vi "Main.vi"() -> ()   [LabVIEW 2017]
doc: "Le programme Main est l'IHM principal du programme MonoSelector. Il controle le sélecteur d'onde de la manipe \"FastFlim\". Il acquit le spectre du laser et permet de positioner le sélecteur ainsi que de choisir la bande passante des ondes lumineuse."
uses:
  Lib IHM Control/MHL Data.ctl
  Lib IHM Control/MHL UI Data.ctl
  <vilib>/vision/Image Controls.llb/IMAQ Image.ctl
  Lib IHM Control/MHL UI Ref.ctl
  Lib IHM Control/Front Panel Status.ctl
  Lib QMH/MessageQueues.lvlib
  Lib Notifier/Notifier.lvlib
  Lib IHM Control/IHM Control.lvlib
  Lib Log/Logging.lvlib
panel:
  in  "Pulse Picker Set":u16(ring) items=["80"=80, "40"=40, "20"=20]
  out "Laser Connection":bool
  out "Camera":T1(plugin-control)
  in  "Integration (ms)":i32=100
  in  "Stop":bool
  in  "View":bool
  in  "LaserON":bool
  out "Power":dbl
  in  "LaserOFF":bool
  out "Pulse Picker":dbl
  in  "Power Set":dbl=480.0
  out "StedFLIM Status":string
  # "Laser"
  # "Camera"
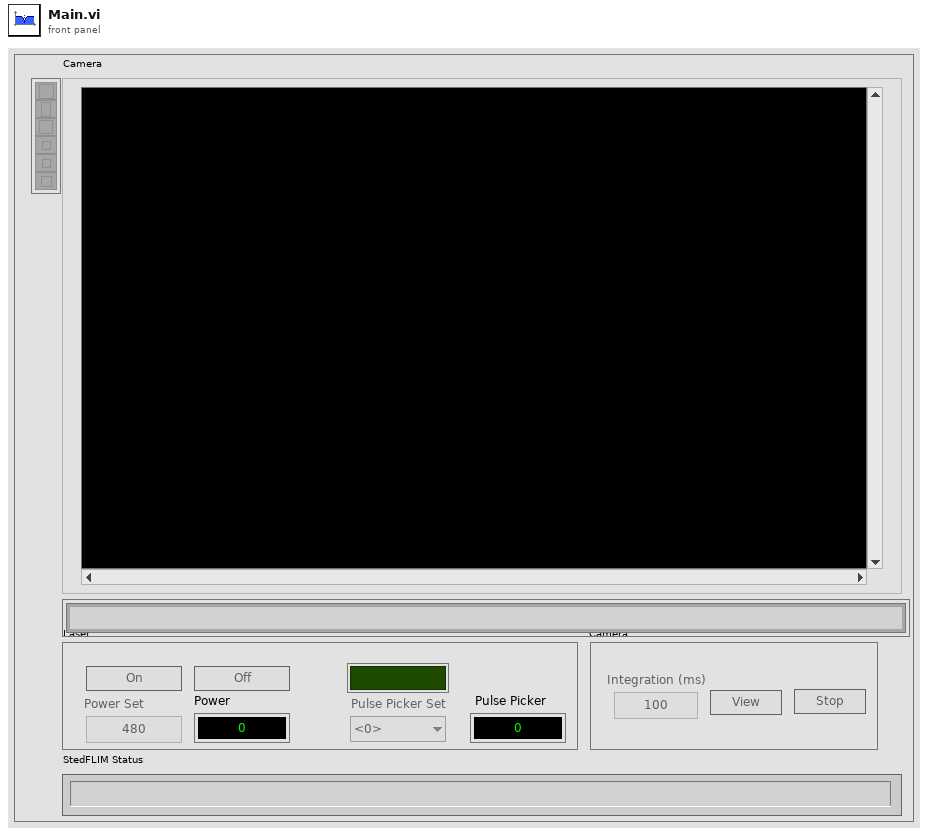
[diagram p1: front panel]
types:
  T1 = typedef "IMAQ Image.ctl" = refnum<image>
  T2 = typedef "MHL Data.ctl" = cluster{"IHM Data":T3, "MHL ref":T4, "Front Panel status":T5}
  T3 = typedef "MHL UI Data.ctl" = cluster{"Integration":i32, "Set Power":dbl, "Power":dbl, "Set Pulse Picke":dbl, "Pulse Picker":dbl, "Status StedFLIM":string, "View":T1, "Laser Connection":bool}
  T4 = typedef "IHM Control.lvlib/MHL UI Ref.ctl" = cluster{"View":refnum<vi>, "Stop":refnum<vi>, "Laser OFF":refnum<vi>, "Laser ON":refnum<vi>, "Integration":refnum<vi>, "SetPower":refnum<vi>, "SetPulsePicker":refnum<vi>}
  T5 = typedef "IHM Control.lvlib/Front Panel Status.ctl" = enum16{"Initialisation", "Enable Laser", "Enable Camera", "Disable Laser", "Disable Camera"}
  T6 = typedef "MessageQueues.lvlib/AllMessageQueue Cluster.ctl" = cluster{"MHL":refnum<queue>, "Recipe":refnum<queue>, "Laser":refnum<queue>, "Laser Controller":refnum<queue>, "Camera":refnum<queue>, "Camera Controller":refnum<queue>, "Manager":refnum<queue>}
  T7 = typedef "Notifier.lvlib/Notifier.ctl" = cluster{"Camera Handshake":refnum<notifier>, "Camera Ctrl Exit":refnum<notifier>, "Camera Exit":refnum<notifier>, "Laser Hanshake":refnum<notifier>, "Laser Ctrl Exit":refnum<notifier>, "Laser Exit":refnum<notifier>}
  T8 = enum16{"open", "replace", "create", "open or create", "replace or create", "replace or create with confirmation"}
  T9 = cluster{"état":bool, "code":i32, "source":string}
  T10 = enum32{"Invalid", "Standard", "Closed", "Hidden", "Minimized", "Maximized"}
  T11 = enum32{"invalid app kind", "Development System", "Run Time System", "Student Edition", "Embedded LabVIEW", "Evaluation", "Custom"}
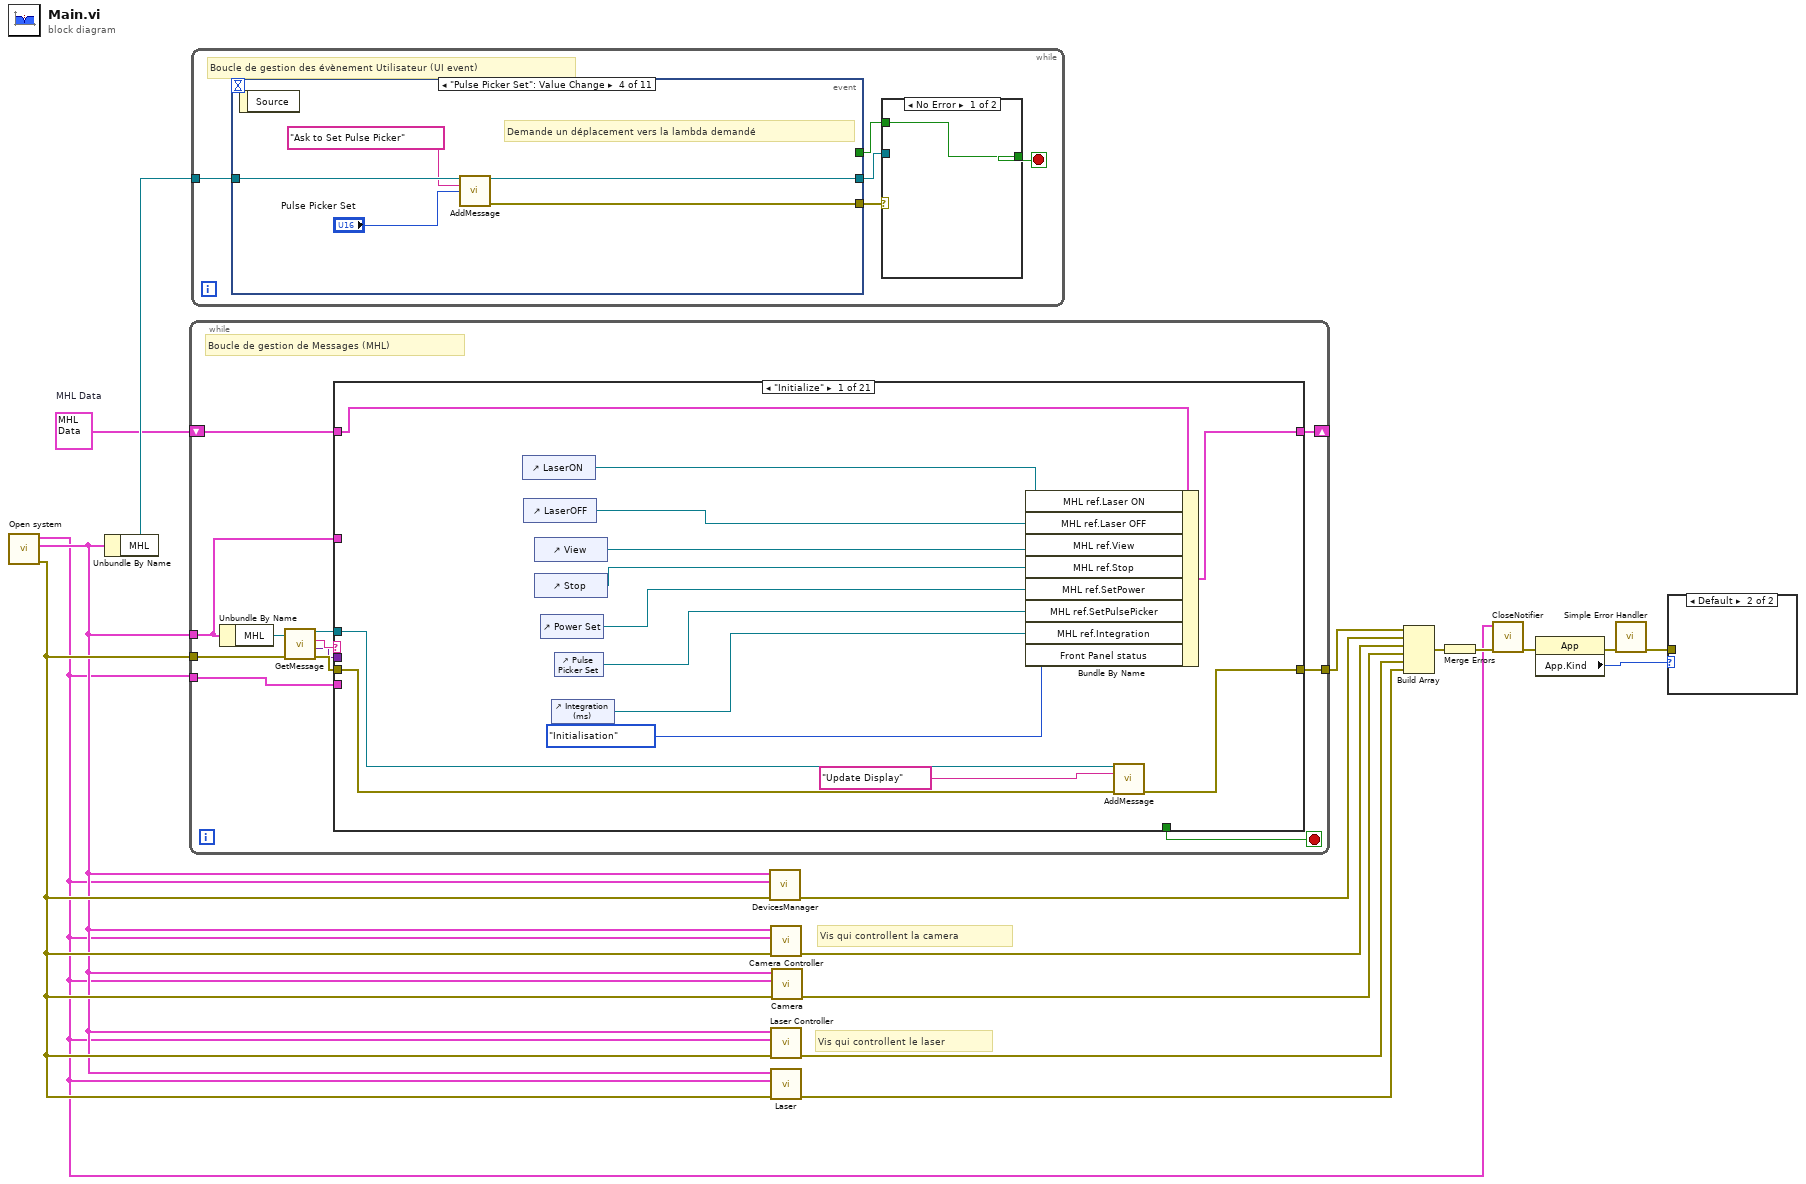
[diagram p0: block diagram]
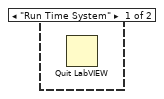
[diagram p2: hidden frame]
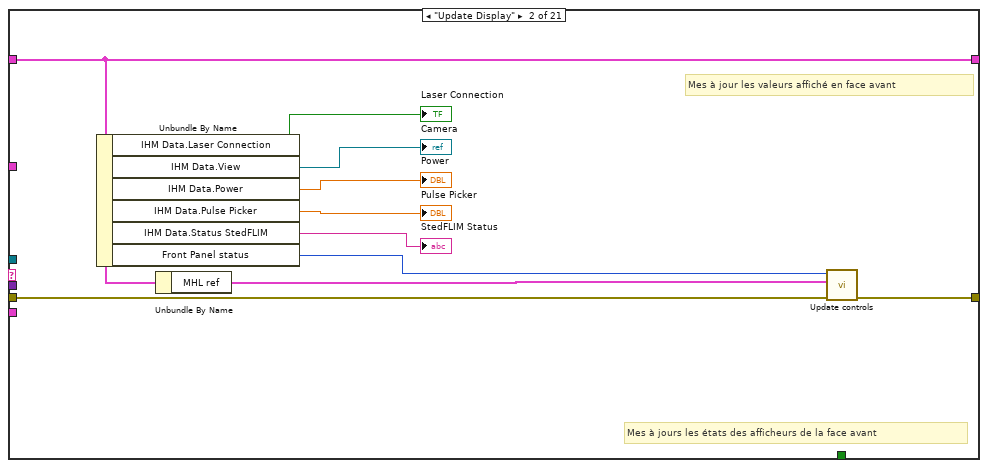
[diagram p3: hidden frame]
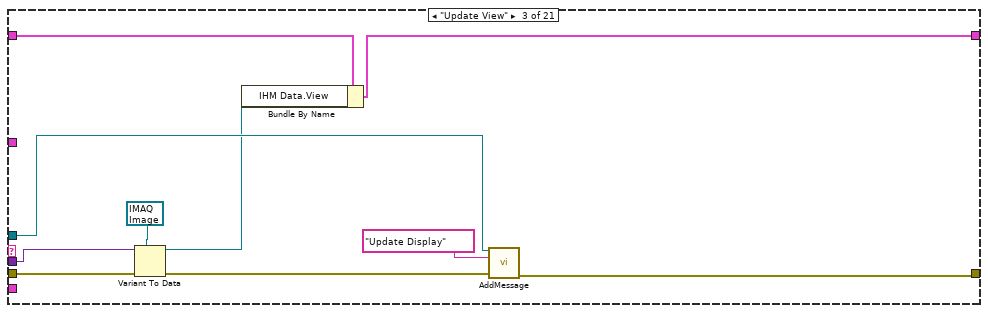
[diagram p4: hidden frame]
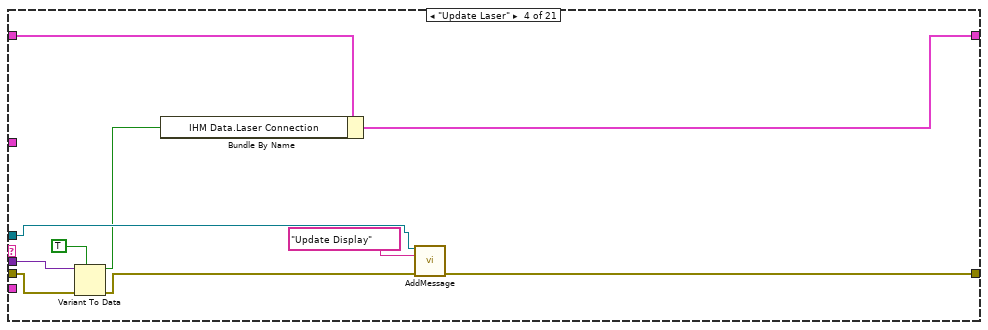
[diagram p5: hidden frame]
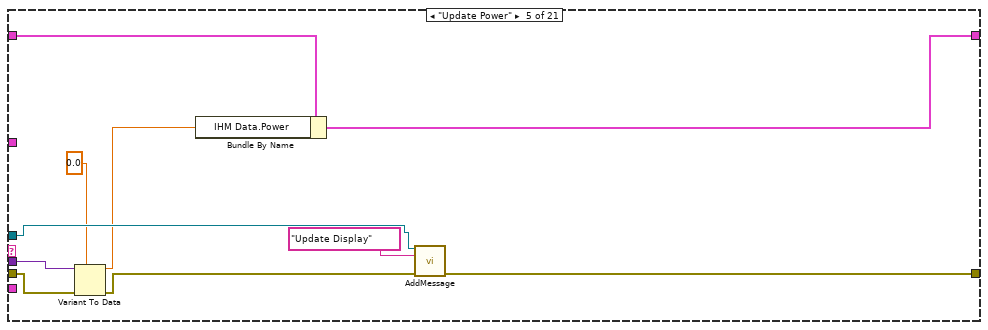
[diagram p6: hidden frame]
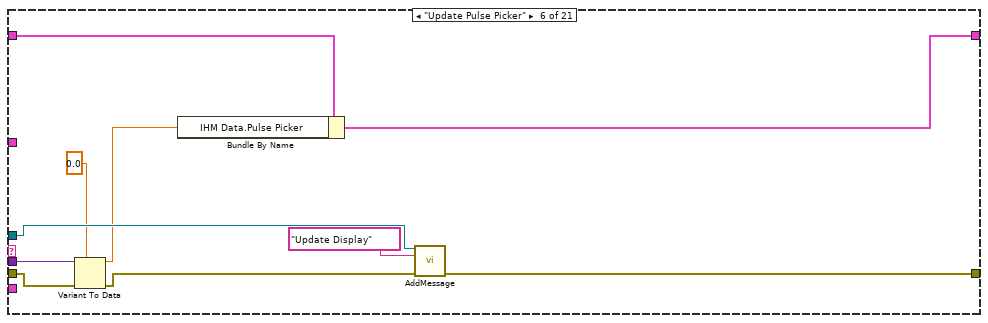
[diagram p7: hidden frame]
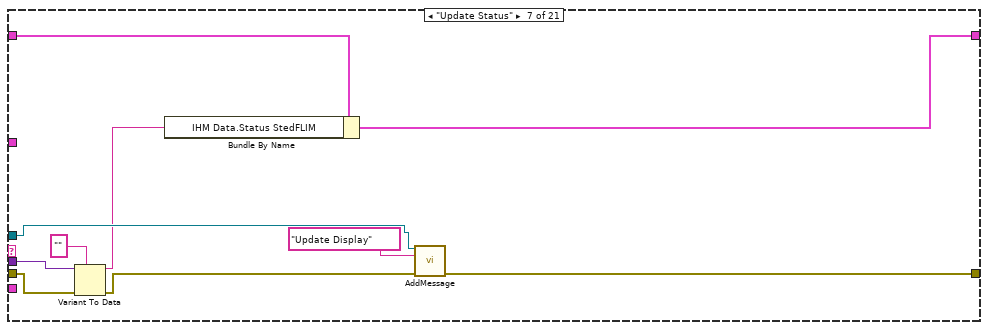
[diagram p8: hidden frame]
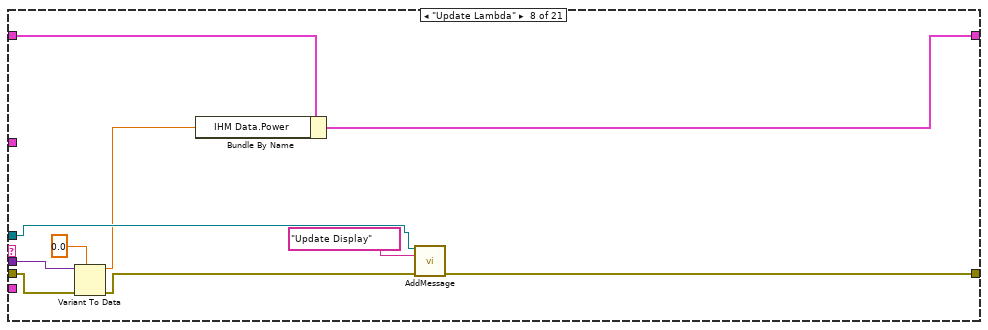
[diagram p9: hidden frame]
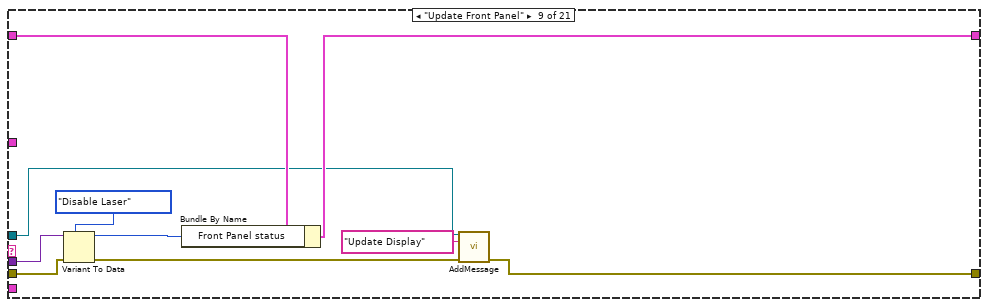
[diagram p10: hidden frame]
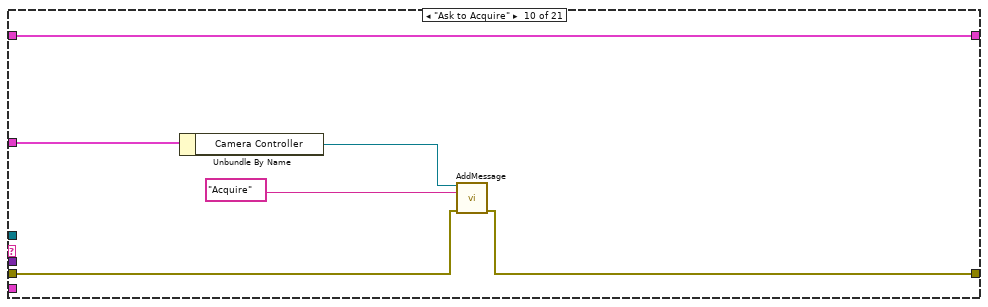
[diagram p11: hidden frame]
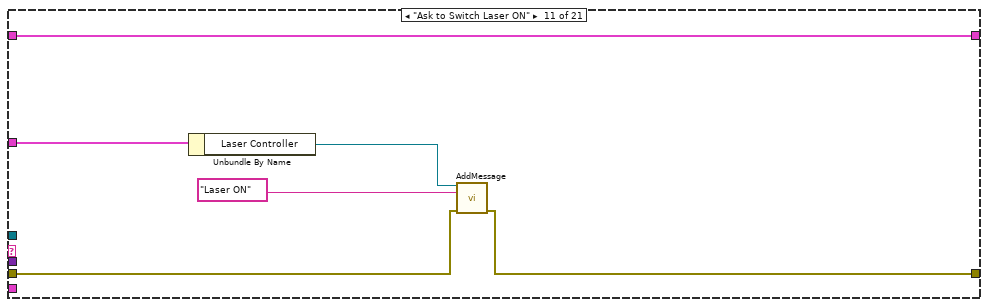
[diagram p12: hidden frame]
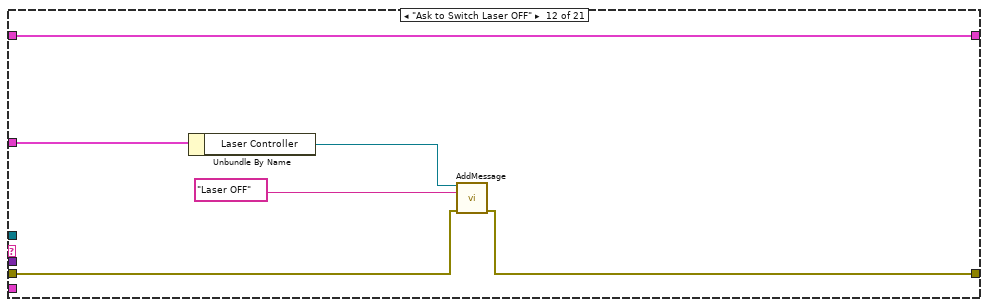
[diagram p13: hidden frame]
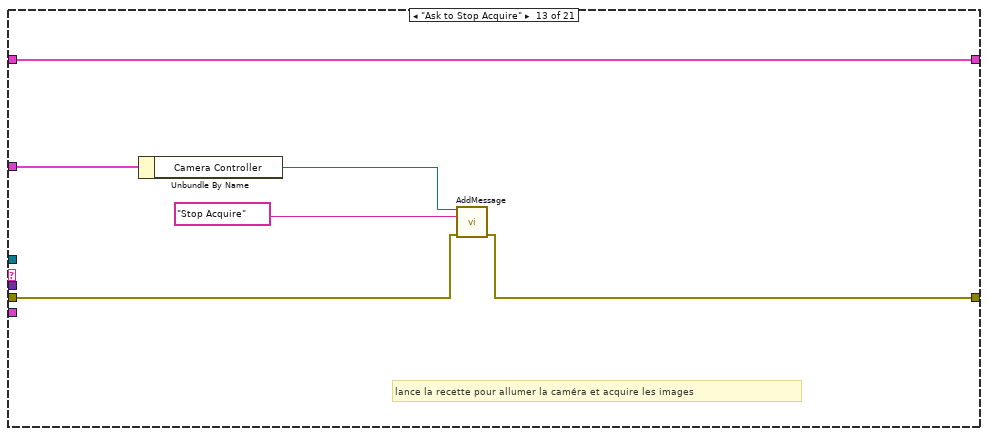
[diagram p14: hidden frame]
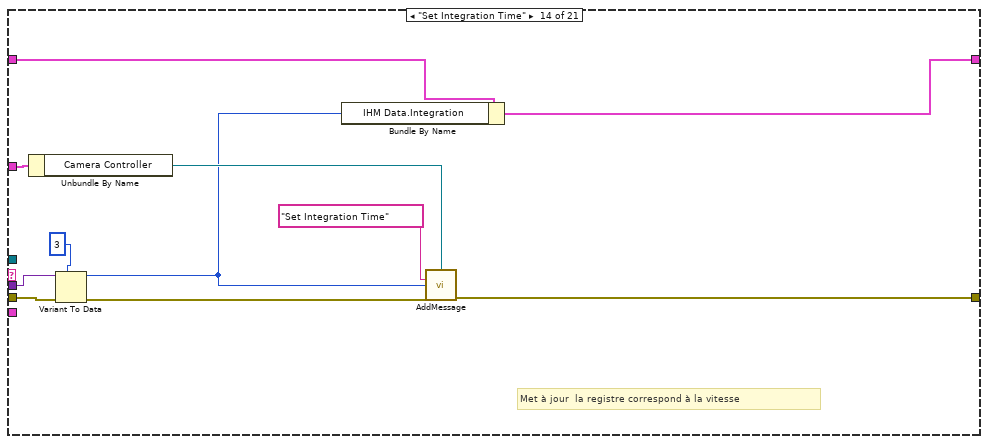
[diagram p15: hidden frame]
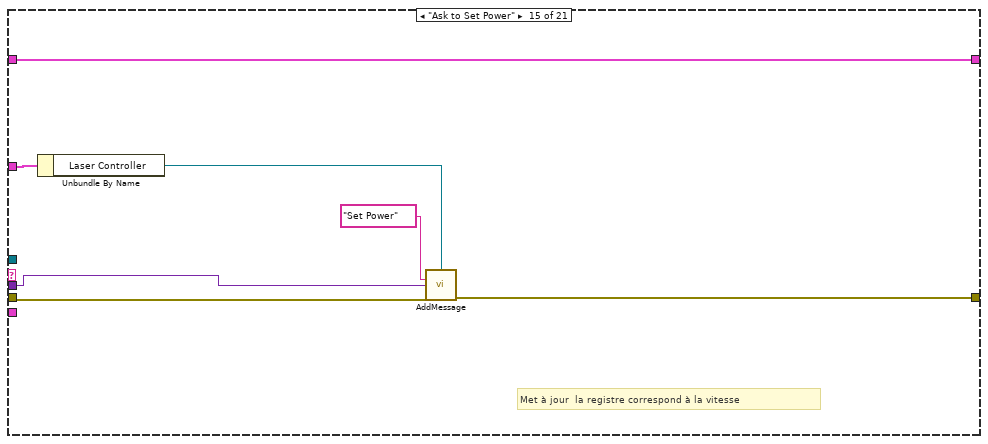
[diagram p16: hidden frame]
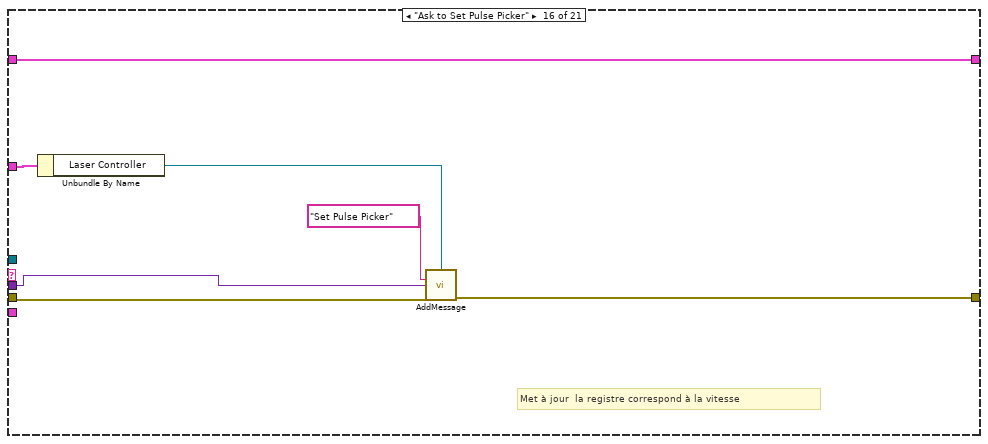
[diagram p17: hidden frame]
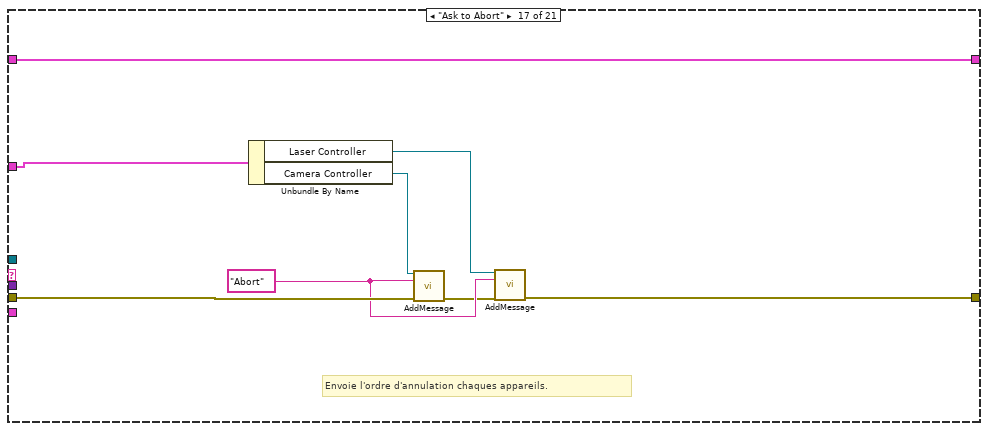
[diagram p18: hidden frame]
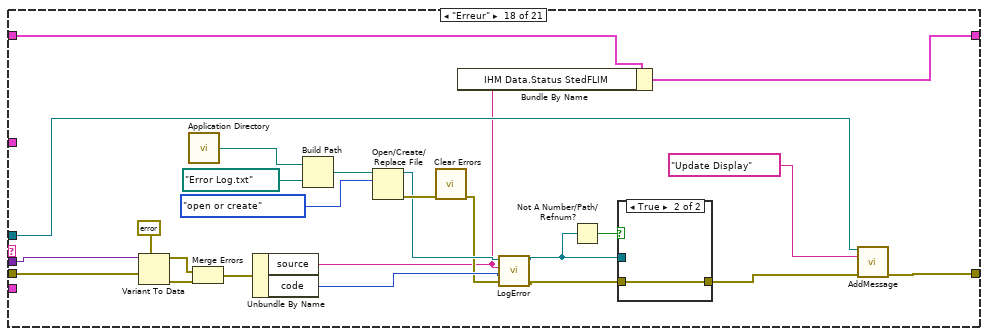
[diagram p19: hidden frame]
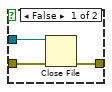
[diagram p20: hidden frame]
diagram:
  w10 = T2 {"IHM Data"={"Integration"=0, "Set Power"=0.0, "Power"=0.0, "Set Pulse Picke"=0.0, "Pulse Picker"=0.0, "Status StedFLIM"="", "View"=refnum, "Laser Connection"=FALSE}, "MHL ref"={"View"=refnum, "Stop"=refnum, "Laser OFF"=refnum, "Laser ON"=refnum, "Integration"=refnum, "SetPower"=refnum, "SetPulsePicker"=refnum}, "Front Panel status"=enum."Initialisation"}  # MHL Data
  # "Vis qui controllent le laser"
  # "Vis qui controllent la camera"
  n1 = call "Open system.vi"() -> ("error out"=w5:errorcluster, "All Message Queue Cluster"=w2:T6, "Notifiers"=w1:T7)  [unwired: 8 in, 1 out]
  n2 = Unbundle By Name(w2) -> ("MHL"=w13:refnum<queue>)
  n3 = while {
    tunnel: w1 -> [w27]
    tunnel: w2 -> [w26]
    shift-right: [w18] -> _
    shift-left: w10 -> [w19]
    tunnel: w5 -> [w24]
    tunnel: [w29] -> w4
    stop <- w28 stop-if-true
    # "Boucle de gestion de Messages (MHL)"
    n4 = Unbundle By Name(w26) -> ("MHL"=w25:refnum<queue>)
    n5 = call "GetMessage.vi"("entrée d'erreur"=w24, "Message queue"=w25) -> ("sortie d'erreur"=w23:errorcluster, "Data"=w20:variant, "Message"=w21:string, "Dup Message Queue"=w22:refnum<queue>)  [unwired: 6 in]
    n6 = case shown="\"Initialize\"" w21 {
      tunnel: w26 -> [_ _ _ _ _ _ _ _ _ w129 w135 w141 w147 w157 w164 w171 w180 _ _ _ w228]
      tunnel: w22 -> [w39 _ w57 w71 w81 w91 w101 w111 w115 _ _ _ _ _ _ _ _ w185 _ w215 _]
      tunnel: w23 -> [w41 w53 w62 w68 w79 w89 w98 w108 w123 w126 w132 w138 w144 w153 w160 w167 w177 w194 w211 w214 w217]
      tunnel: [w40 w52 w58 w72 w82 w92 w102 w112 w116 w125 w131 w137 w143 w158 w165 w172 w173 w186 w211 w213 w220] -> w29
      tunnel: [_ _ _ _ _ _ _ _ _ _ _ _ _ _ _ _ _ _ _ TRUE _] -> w28
      tunnel: w27 -> [_ _ _ _ _ _ _ _ _ _ _ _ _ _ _ _ _ _ _ _ _]
      tunnel: w20 -> [_ _ w61 w70 w80 w90 w100 w110 w122 _ _ _ _ w151 w161 w168 _ w193 _ _ _]
      tunnel: w19 -> [w43 w50 w63 w66 w77 w87 w96 w106 w120 w124 w130 w136 w142 w154 w159 w166 w178 w184 w209 w212 w227]
      tunnel: [w42 w50 w56 w65 w76 w86 w95 w105 w118 w124 w130 w136 w142 w148 w159 w166 w178 w181 w209 w212 w227] -> w18
      frame "Initialize" {
        n7 = control-ref of="LaserON"() -> (w31:refnum<vi>)
        n8 = control-ref of="LaserOFF"() -> (w32:refnum<vi>)
        n9 = control-ref of="View"() -> (w33:refnum<vi>)
        n10 = control-ref of="Stop"() -> (w34:refnum<vi>)
        n11 = control-ref of="Power Set"() -> (w35:refnum<vi>)
        n12 = control-ref of="Integration (ms)"() -> (w36:refnum<vi>)
        n13 = control-ref of="Pulse Picker Set"() -> (w30:refnum<vi>)
        n14 = Bundle By Name(cluster=w43, "MHL ref.Laser ON"=w31, "MHL ref.Laser OFF"=w32, "MHL ref.View"=w33, "MHL ref.Stop"=w34, "MHL ref.SetPower"=w35, "MHL ref.SetPulsePicker"=w30, "MHL ref.Integration"=w36, "Front Panel status"=Front_Panel_Status."Initialisation") -> (w42:T2)
        n15 = call "AddMessage.vi"("Message queue"=w39, "Message"="Update Display", "entrée d'erreur (pas d'erreur)"=w41) -> ("error out"=w40:errorcluster)  [unwired: 11 in, 1 out]
      }
      frame "Update Display" {
        # "Mes à jours les états des afficheurs de la face avant"
        # "Mes à jour les valeurs affiché en face avant"
        n16 = Unbundle By Name(w50) -> ("IHM Data.Laser Connection"=→"Laser Connection":bool, "IHM Data.View"=→"Camera":T1, "IHM Data.Power"=→"Power":dbl, "IHM Data.Pulse Picker"=→"Pulse Picker":dbl, "IHM Data.Status StedFLIM"=→"StedFLIM Status":string, "Front Panel status"=w49:T5)
        n17 = Unbundle By Name(w50) -> ("MHL ref"=w51:T4)
        n18 = call "Update controls.vi"("error in (no error)"=w53, "IHM Data refnum"=w51, "Front Panel status"=w49) -> ("error out"=w52:errorcluster)  [unwired: 8 in]
      }
      frame "Update View" {
        n19 = Variant To Data(error in=w62, type=T1 refnum ("IHM Data.View"), Variant=w61) -> (data=w54:T1, error out=w59:errorcluster)
        n20 = Bundle By Name(cluster=w63, "IHM Data.View"=w54) -> (w56:T2)
        n21 = call "AddMessage.vi"("Message queue"=w57, "Message"="Update Display", "entrée d'erreur (pas d'erreur)"=w59) -> ("error out"=w58:errorcluster)  [unwired: 11 in, 1 out]
      }
      frame "Update Laser" {
        n22 = Variant To Data(error in=w68, type=TRUE, Variant=w70) -> (data=w64:bool, error out=w67:errorcluster)
        n23 = Bundle By Name(cluster=w66, "IHM Data.Laser Connection"=w64) -> (w65:T2)
        n24 = call "AddMessage.vi"("Message queue"=w71, "Message"="Update Display", "entrée d'erreur (pas d'erreur)"=w67) -> ("error out"=w72:errorcluster)  [unwired: 11 in, 1 out]
      }
      frame "Update Power" {
        n25 = Variant To Data(error in=w79, type=0.0, Variant=w80) -> (data=w74:dbl, error out=w78:errorcluster)
        n26 = Bundle By Name(cluster=w77, "IHM Data.Power"=w74) -> (w76:T2)
        n27 = call "AddMessage.vi"("Message queue"=w81, "Message"="Update Display", "entrée d'erreur (pas d'erreur)"=w78) -> ("error out"=w82:errorcluster)  [unwired: 11 in, 1 out]
      }
      frame "Update Pulse Picker" {
        n28 = Variant To Data(error in=w89, type=0.0, Variant=w90) -> (data=w84:dbl, error out=w88:errorcluster)
        n29 = Bundle By Name(cluster=w87, "IHM Data.Pulse Picker"=w84) -> (w86:T2)
        n30 = call "AddMessage.vi"("Message queue"=w91, "Message"="Update Display", "entrée d'erreur (pas d'erreur)"=w88) -> ("error out"=w92:errorcluster)  [unwired: 11 in, 1 out]
      }
      frame "Update Status" {
        n31 = Variant To Data(error in=w98, type="", Variant=w100) -> (data=w94:string, error out=w97:errorcluster)
        n32 = Bundle By Name(cluster=w96, "IHM Data.Status StedFLIM"=w94) -> (w95:T2)
        n33 = call "AddMessage.vi"("Message queue"=w101, "Message"="Update Display", "entrée d'erreur (pas d'erreur)"=w97) -> ("error out"=w102:errorcluster)  [unwired: 11 in, 1 out]
      }
      frame "Update Lambda" {
        n34 = Variant To Data(error in=w108, type=0.0, Variant=w110) -> (data=w104:dbl, error out=w107:errorcluster)
        n35 = Bundle By Name(cluster=w106, "IHM Data.Power"=w104) -> (w105:T2)
        n36 = call "AddMessage.vi"("Message queue"=w111, "Message"="Update Display", "entrée d'erreur (pas d'erreur)"=w107) -> ("error out"=w112:errorcluster)  [unwired: 11 in, 1 out]
      }
      frame "Update Front Panel" {
        n37 = Variant To Data(error in=w123, type=Front_Panel_Status."Disable Laser" ("Front Panel status"), Variant=w122) -> (data=w119:T5, error out=w117:errorcluster)
        n38 = Bundle By Name(cluster=w120, "Front Panel status"=w119) -> (w118:T2)
        n39 = call "AddMessage.vi"("Message queue"=w115, "Message"="Update Display", "entrée d'erreur (pas d'erreur)"=w117) -> ("error out"=w116:errorcluster)  [unwired: 11 in, 1 out]
      }
      frame "Ask to Acquire" {
        n40 = Unbundle By Name(w129) -> ("Camera Controller"=w128:refnum<queue>)
        n41 = call "AddMessage.vi"("Message queue"=w128, "Message"="Acquire", "entrée d'erreur (pas d'erreur)"=w126) -> ("error out"=w125:errorcluster)  [unwired: 11 in, 1 out]
      }
      frame "Ask to Switch Laser ON" {
        n42 = Unbundle By Name(w135) -> ("Laser Controller"=w134:refnum<queue>)
        n43 = call "AddMessage.vi"("Message queue"=w134, "Message"="Laser ON", "entrée d'erreur (pas d'erreur)"=w132) -> ("error out"=w131:errorcluster)  [unwired: 11 in, 1 out]
      }
      frame "Ask to Switch Laser OFF" {
        n44 = Unbundle By Name(w141) -> ("Laser Controller"=w140:refnum<queue>)
        n45 = call "AddMessage.vi"("Message queue"=w140, "Message"="Laser OFF", "entrée d'erreur (pas d'erreur)"=w138) -> ("error out"=w137:errorcluster)  [unwired: 11 in, 1 out]
      }
      frame "Ask to Stop Acquire" {
        # "lance la recette pour allumer la caméra et acquire les images"
        n46 = Unbundle By Name(w147) -> ("Camera Controller"=w146:refnum<queue>)
        n47 = call "AddMessage.vi"("Message queue"=w146, "Message"="Stop Acquire", "entrée d'erreur (pas d'erreur)"=w144) -> ("error out"=w143:errorcluster)  [unwired: 11 in, 1 out]
      }
      frame "Set Integration Time" {
        # "Met à jour  la registre correspond à la vitesse"
        n48 = Unbundle By Name(w157) -> ("Camera Controller"=w156:refnum<queue>)
        n49 = Variant To Data(error in=w153, type=3 ("Integration (ms)"), Variant=w151) -> (data=w149:i32, error out=w152:errorcluster)
        n50 = Bundle By Name(cluster=w154, "IHM Data.Integration"=w149) -> (w148:T2)
        n51 = call "AddMessage.vi"("Message queue"=w156, "Message"="Set Integration Time", "Data"=w149, "entrée d'erreur (pas d'erreur)"=w152) -> ("error out"=w158:errorcluster)  [unwired: 10 in, 1 out]
      }
      frame "Ask to Set Power" {
        # "Met à jour  la registre correspond à la vitesse"
        n52 = Unbundle By Name(w164) -> ("Laser Controller"=w163:refnum<queue>)
        n53 = call "AddMessage.vi"("Message queue"=w163, "Message"="Set Power", "Data"=w161, "entrée d'erreur (pas d'erreur)"=w160) -> ("error out"=w165:errorcluster)  [unwired: 10 in, 1 out]
      }
      frame "Ask to Set Pulse Picker" {
        # "Met à jour  la registre correspond à la vitesse"
        n54 = Unbundle By Name(w171) -> ("Laser Controller"=w170:refnum<queue>)
        n55 = call "AddMessage.vi"("Message queue"=w170, "Message"="Set Pulse Picker", "Data"=w168, "entrée d'erreur (pas d'erreur)"=w167) -> ("error out"=w172:errorcluster)  [unwired: 10 in, 1 out]
      }
      frame "Ask to Abort" {
        w175 = "Abort" ("Message")
        # "Envoie l'ordre d'annulation chaques appareils."
        n56 = Unbundle By Name(w180) -> ("Laser Controller"=w176:refnum<queue>, "Camera Controller"=w179:refnum<queue>)
        n57 = call "AddMessage.vi"("Message queue"=w179, "Message"=w175, "entrée d'erreur (pas d'erreur)"=w177) -> ("error out"=w174:errorcluster)  [unwired: 11 in, 1 out]
        n58 = call "AddMessage.vi"("Message queue"=w176, "Message"=w175, "entrée d'erreur (pas d'erreur)"=w174) -> ("error out"=w173:errorcluster)  [unwired: 11 in, 1 out]
      }
      frame "Erreur" {
        n59 = Variant To Data(error in=w194, type=T9 {"état"=FALSE, "code"=0, "source"=""} ("sortie d'erreur"), Variant=w193) -> (data=w202:T9, error out=w203:errorcluster)
        n60 = call <vilib>:"Application Directory.vi"() -> ("Application Directory"=w200:path)
        n61 = Merge Errors(w202, w203) -> (w201:errorcluster)
        n62 = Unbundle By Name(w201) -> ("source"=w183:string, "code"=w190:i32)
        n63 = Build Path(base path=w200, name or relative path=path "Error Log.txt") -> (appended path=w199:path)
        n64 = Open/Create/Replace File(file path (use dialog)=w199, operation (0:open)=T8."open or create" ("opération (0 : open)")) -> (refnum out=w192:refnum<file>, error out=w195:errorcluster)  [unwired: 4 in, 1 out]
        n65 = call <vilib>:"Clear Errors.vi"("error in (no error)"=w195) -> ("error out"=w189:errorcluster)  [unwired: 5 in, 1 out]
        n66 = Bundle By Name(cluster=w184, "IHM Data.Status StedFLIM"=w183) -> (w181:T2)
        n67 = call "LogError.vi"("entrée d'erreur"=w189, "Code"=w190, "Source"=w183, "Error log refnum In"=w192) -> ("error out"=w188:errorcluster, "Error log refnum out"=w191:refnum<file>)  [unwired: 6 in]
        n68 = Not A Number/Path/Refnum?(number/path/refnum=w191) -> (NaN/Path/Refnum?=w196:bool)
        n69 = case shown="True" w196 {
          tunnel: w188 -> [w207 w208]
          tunnel: w191 -> [w206 _]
          tunnel: [w205 w208] -> w187
          frame False {
            n70 = Close File(refnum=w206, error in=w207) -> (error out=w205:errorcluster)  [unwired: 1 out]
          }
          frame True {
          }
        }
        n71 = call "AddMessage.vi"("Message queue"=w185, "Message"="Update Display", "entrée d'erreur (pas d'erreur)"=w187) -> ("error out"=w186:errorcluster)  [unwired: 11 in, 1 out]
      }
      frame Default {
        n72 = One Button Dialog(message="Warning : Message erroné ou erreur dans le MHL") -> ()  [unwired: 1 in, 1 out]
      }
      frame "Quit" {
        # "Libère la pile MHL et stop la boucle"
        n73 = Release Queue(queue=w215, error in (no error)=w214) -> (error out=w213:errorcluster)  [unwired: 1 in, 2 out]
      }
      frame "Initiate Stop" {
        w218 = "Exit" ("Message")
        # "Envoie un message d'arrête à tous les controleur.\nPuis demande d'attendre jusqu'à ce que chaque appareils soit arrêtés"
        n74 = Unbundle By Name(w228) -> ("MHL"=w219:refnum<queue>, "Laser Controller"=w226:refnum<queue>, "Camera Controller"=w225:refnum<queue>, "Manager"=w224:refnum<queue>)
        n75 = call "AddMessage.vi"("Message queue"=w225, "Message"=w218, "entrée d'erreur (pas d'erreur)"=w217) -> ("error out"=w222:errorcluster)  [unwired: 11 in, 1 out]
        n76 = call "AddMessage.vi"("Message queue"=w224, "Message"=w218, "entrée d'erreur (pas d'erreur)"=w217) -> ("error out"=w221:errorcluster)  [unwired: 11 in, 1 out]
        n77 = call "AddMessage.vi"("Message queue"=w226, "Message"=w218, "entrée d'erreur (pas d'erreur)"=w217) -> ("error out"=w223:errorcluster)  [unwired: 11 in, 1 out]
        n78 = Merge Errors(w223, w222, w221) -> (w220:errorcluster)
        n79 = case shown="No Error" w220 {
          selector: w220 -> [w229 _]
          tunnel: w219 -> [w231 _]
          frame No Error {
            n80 = call "AddMessage.vi"("Message queue"=w231, "Message"="Quit", "entrée d'erreur (pas d'erreur)"=w229) -> ()  [unwired: 11 in, 2 out]
          }
          frame Error {
          }
        }
      }
    }
  }
  n81 = while {
    tunnel: w13 -> [w236]
    stop <- w233 stop-if-true
    # "Boucle de gestion des évènement Utilisateur (UI event)"
    n82 = event shown="[3] \"Pulse Picker Set\": Value Change" {
      selector: _ -> [_ _ _ _ _ _ _ _ _ _ _]
      dyn-events: _ -> [_ _ _ _ _ _ _ _ _ _ _]
      timeout: _ -> [_ _ _ _ _ _ _ _ _ _ _]
      tunnel: w236 -> [_ w242 w250 w255 w259 w282 w288 w292 w297 w302 w307]
      tunnel: [_ w243 w247 w252 w257 w279 w285 w289 w294 w299 w305] -> w235
      tunnel: [_ TRUE ("Message Priority ?") _ _ w256 TRUE ("Message Priority ?") _ _ _ _ _] -> w234
      tunnel: [_ w244 w248 w253 w258 w280 w286 w290 w295 w300 w306] -> w232
      event Timeout {
        n83 = event-data() -> ()  [unwired: 1 in, 2 out]
      }
      event Application Instance Close {
        n84 = event-data() -> ()  [unwired: 1 in, 1 out]
        n85 = call "AddMessage.vi"("Message queue"=w242, "Message"="Initiate Stop") -> ("Dup Message queue"=w244:refnum<queue>, "error out"=w243:errorcluster)  [unwired: 12 in]
      }
      event "Power Set": Value Change {
        # "Demande un déplacement vers la lambda demandé"
        n86 = event-data() -> ()  [unwired: 1 in, 1 out]
        n87 = call "AddMessage.vi"("Message queue"=w250, "Message"="Ask to Set Power", "Data"="Power Set") -> ("Dup Message queue"=w248:refnum<queue>, "error out"=w247:errorcluster)  [unwired: 11 in]
      }
      event "Pulse Picker Set": Value Change {
        # "Demande un déplacement vers la lambda demandé"
        n88 = event-data() -> ()  [unwired: 1 in, 1 out]
        n89 = call "AddMessage.vi"("Message queue"=w255, "Message"="Ask to Set Pulse Picker", "Data"="Pulse Picker Set") -> ("Dup Message queue"=w253:refnum<queue>, "error out"=w252:errorcluster)  [unwired: 11 in]
      }
      event Menu Selection (User) {
        n90 = event-data() -> ("ItemTag"=w260:string)  [unwired: 1 in]
        n91 = case shown="\"Camera\"" w260 {
          tunnel: w259 -> [w261 w265 w269 w273 w277]
          tunnel: [w261 w265 w269 w273 w276] -> w258
          tunnel: [_ _ _ _ w275] -> w257
          tunnel: [_ _ _ _ TRUE ("Message Priority ?")] -> w256
          frame Default {
          }
          frame "Camera" {
            # "Ouvre la FA du spectro"
            n92 = vi-ref "Camera.vi"() -> (w262:refnum<vi>)
            n93 = invoke class="VI" method="FP.Open"(reference=w262, "Activate"=TRUE ("Activate?"), "State"=T10."Standard") -> ()  [unwired: 2 in, 5 out]
          }
          frame "Manager" {
            # "Ouvre la FA du spectro"
            n94 = vi-ref "DevicesManager.vi"() -> (w266:refnum<vi>)
            n95 = invoke class="VI" method="FP.Open"(reference=w266, "Activate"=TRUE ("Activate?"), "State"=T10."Standard") -> ()  [unwired: 2 in, 5 out]
          }
          frame "Laser" {
            # "Ouvre la FA du Slit"
            n96 = vi-ref "Laser.vi"() -> (w272:refnum<vi>)
            n97 = invoke class="VI" method="FP.Open"(reference=w272, "Activate"=TRUE ("Activate?"), "State"=T10."Standard") -> ()  [unwired: 2 in, 5 out]
          }
          frame "Quit" {
            n98 = call "AddMessage.vi"("Message queue"=w277, "Message"="Initiate Stop") -> ("Dup Message queue"=w276:refnum<queue>, "error out"=w275:errorcluster)  [unwired: 12 in]
          }
        }
      }
      event Panel Close {
        n99 = event-data() -> ()  [unwired: 1 in, 4 out]
        n100 = call "AddMessage.vi"("Message queue"=w282, "Message"="Initiate Stop", "Message Priority ?"=TRUE) -> ("Dup Message queue"=w280:refnum<queue>, "error out"=w279:errorcluster)  [unwired: 11 in]
      }
      event "View": Value Change {
        # "demande le déplacement du moteur à vers le position mémorisée dans Reg X"
        n101 = event-data() -> ()  [unwired: 1 in, 1 out]
        n102 = call "AddMessage.vi"("Message queue"=w288, "Message"="Ask to Acquire") -> ("Dup Message queue"=w286:refnum<queue>, "error out"=w285:errorcluster)  [unwired: 12 in]
      }
      event "Stop": Value Change {
        # "demande le déplacement du moteur à vers le position mémorisée dans Reg X"
        n103 = event-data() -> ()  [unwired: 1 in, 1 out]
        n104 = call "AddMessage.vi"("Message queue"=w292, "Message"="Ask to Stop Acquire") -> ("Dup Message queue"=w290:refnum<queue>, "error out"=w289:errorcluster)  [unwired: 12 in]
      }
      event "LaserON": Value Change {
        # "demande le déplacement du moteur à vers le position mémorisée dans Reg X"
        n105 = event-data() -> ()  [unwired: 1 in, 6 out]
        n106 = call "AddMessage.vi"("Message queue"=w297, "Message"="Ask to Switch Laser ON", "Data"=TRUE ("Dlambda +")) -> ("Dup Message queue"=w295:refnum<queue>, "error out"=w294:errorcluster)  [unwired: 11 in]
      }
      event "LaserOFF": Value Change {
        # "demande le déplacement du moteur à vers le position mémorisée dans Reg X"
        n107 = event-data() -> ()  [unwired: 1 in, 6 out]
        n108 = call "AddMessage.vi"("Message queue"=w302, "Message"="Ask to Switch Laser OFF", "Data"=FALSE ("Dlambda +")) -> ("Dup Message queue"=w300:refnum<queue>, "error out"=w299:errorcluster)  [unwired: 11 in]
      }
      event "Integration (ms)": Value Change {
        n109 = event-data() -> ()  [unwired: 1 in, 1 out]
        n110 = call "AddMessage.vi"("Message queue"=w307, "Message"="Set Integration Time", "Data"="Integration (ms)") -> ("Dup Message queue"=w306:refnum<queue>, "error out"=w305:errorcluster)  [unwired: 11 in]
      }
    }
    n111 = case shown="No Error" w235 {
      tunnel: [w237 TRUE ("Message Priority ?")] -> w233
      tunnel: w234 -> [w237 _]
      tunnel: w232 -> [_ w239]
      frame No Error {
      }
      frame Error {
        # "une erreur ferme \nla MHL et stop la boucle\névènementielle"
        n112 = call "AddMessage.vi"("Message queue"=w239, "Message"="Exit") -> ()  [unwired: 12 in, 2 out]
      }
    }
  }
  n113 = call "DevicesManager.vi"("error in (no error)"=w5, "Notifiers"=w1, "All Message Queue Cluster"=w2) -> ("error out"=w3:errorcluster)  [unwired: 8 in]
  n114 = call "Camera Controller.vi"("error in (no error)"=w5, "Notifiers"=w1, "All Message Queue Cluster"=w2) -> ("error out"=w9:errorcluster)  [unwired: 8 in]
  n115 = call "Laser Controller.vi"("error in (no error)"=w5, "Notifiers"=w1, "All Message Queue Cluster"=w2) -> ("error out"=w7:errorcluster)  [unwired: 8 in]
  n116 = call "Laser.vi"("error in (no error)"=w5, "Notifiers"=w1, "All Message Queue Cluster"=w2) -> ("error out"=w6:errorcluster)  [unwired: 8 in]
  n117 = call "Camera.vi"("error in (no error)"=w5, "Notifiers"=w1, "All Message Queue Cluster"=w2) -> ("error out"=w8:errorcluster)  [unwired: 8 in]
  n118 = Build Array(w4, w3, w9, w8, w7, w6) -> (w17:errorcluster[])
  n119 = Merge Errors(w17) -> (w12:errorcluster)
  n120 = call "CloseNotifier.vi"("entrée d'erreur"=w12, "Notifiers"=w1) -> ("error out"=w11:errorcluster)  [unwired: 9 in]
  n121 = property class="App"(error in=w11) -> (error out=w15:errorcluster, "App.Kind"=w16:T11)  [unwired: 1 in, 1 out]
  n122 = call <vilib>:"Simple Error Handler.vi"("error in (no error)"=w15) -> ("error out"=w14:errorcluster)  [unwired: 4 in, 4 out]
  n123 = case shown="Default" w16 {
    tunnel: w14 -> [_ _]
    frame "Run Time System" {
      n124 = Quit LabVIEW() -> ()  [unwired: 1 in]
    }
    frame Default {
    }
  }
